vi "Teleop.vi"(10 "Match Info":T1={"Autonomous Elapsed Seconds"=0.0, "TeleOp Elapsed Seconds"=0.0, "Disabled Elapsed Seconds"=0.0, "Visited Autonomous"=FALSE, "Visited TeleOp"=FALSE, "Visited Disabled"=FALSE, "Autonomous Settings"={"Autonomous Style"=enum."Independent", "VI Refnum"=refnum}}, 11 "Call Context":T2) -> ()   [LabVIEW 2016]
doc: "This VI is called for each TeleOp packet received from the DS where the robot is not disabled. It is often used to read from the joysticks and update I/O or to update setpoints for timed control loops. It should complete and return within 20 milliseconds or it may miss DS packets."
uses:
  <vilib>/Rock Robotics/WPI/DriverStation/WPI_DriverStationDerivedRobotMode.ctl
  <vilib>/Rock Robotics/WPI/DriverStation/WPI_DriverStationMatch Info.ctl
  <vilib>/Rock Robotics/WPI/Utilities/WPI_GetSetVariantRefNum.vi
  <vilib>/Rock Robotics/Network Tables/NT Write Boolean Array.vi
  <vilib>/Rock Robotics/Network Tables/NT Write Numeric Array.vi
  <vilib>/Rock Robotics/Network Tables/NT Read Boolean.vi
  <vilib>/Rock Robotics/Network Tables/NT Read Number.vi
  <vilib>/Rock Robotics/Network Tables/NT Write Boolean.vi
  <vilib>/Rock Robotics/Network Tables/NT Write Number.vi
panel:
  out "Difference":dbl(knob) scale=0.0..50.0
  in  "Reset Counters":bool
  out "Right Wheel Sensor Count":dbl
  out "Left Wheel Sensor Count":dbl
  out "Low Switch":bool
  out "High Switch":bool
  out "POT Sensor Meter":dbl(knob) scale=78.0..98.0
  out "POT Sensor Value":dbl
  out "Sample Slider 0":dbl(slide) scale=0.0..5.0
  out "Sample Boolean 1":bool
  out "Sample Boolean 0":bool
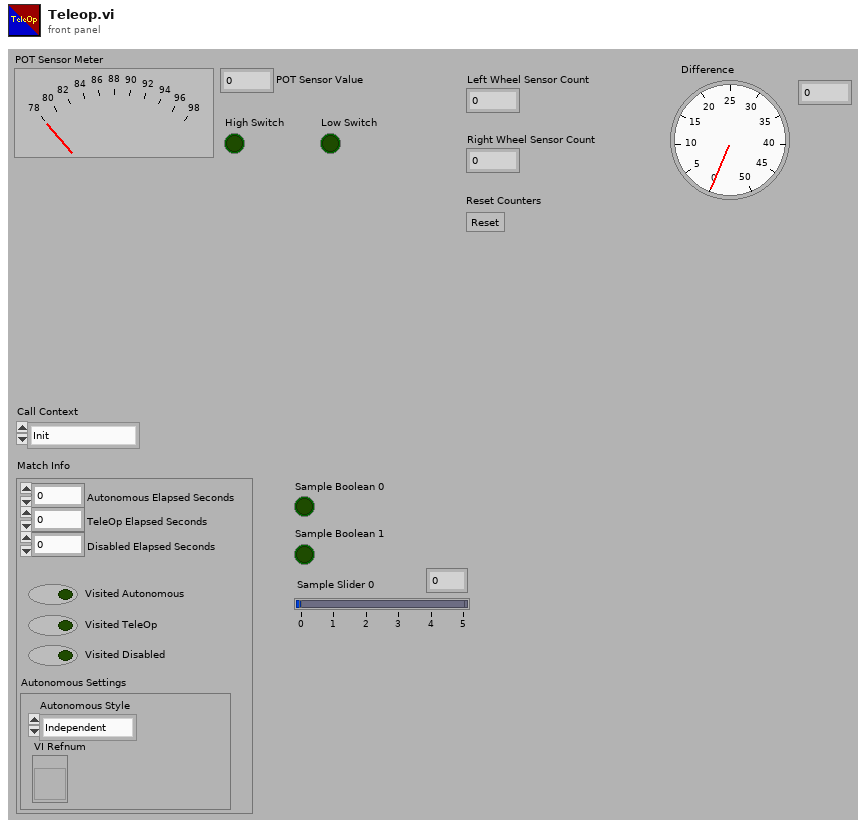
[diagram p1: front panel]
types:
  T1 = typedef "WPI_DriverStationMatch Info.ctl" = cluster{"Autonomous Elapsed Seconds":dbl, "TeleOp Elapsed Seconds":dbl, "Disabled Elapsed Seconds":dbl, "Visited Autonomous":bool, "Visited TeleOp":bool, "Visited Disabled":bool, "Autonomous Settings":cluster{"Autonomous Style":enum16{"Iterative", "Independent"}, "VI Refnum":refnum<vi>}}
  T2 = typedef "WPI_DriverStationDerivedRobotMode.ctl" = enum16{"Init", "Execute", "Stop"}
  T3 = typedef "WPI_JoystickDevRef.ctl" = cluster{"Device":T4}
  T4 = typedef "WPI_JoystickDeviceEnum.ctl" = enum16{"USB 0", "USB 1", "USB 2", "USB 3", "USB 4", "USB 5"}
  T5 = typedef "WPI_SwitchDevRef.ctl" = cluster{"DevStatus":errorcluster, "DIO Channel":T6, "CntIndex":T7, "Normally Closed":bool}
  T6 = typedef "FPGA_DIOChannel.ctl" = enum8{"DIO 0", "DIO 1", "DIO 2", "DIO 3", "DIO 4", "DIO 5", "DIO 6", "DIO 7", "DIO 8", "DIO 9", "DIO MXP 0", "DIO MXP 1", "DIO MXP 2", "DIO MXP 3", "DIO MXP 4", "DIO MXP 5", "DIO MXP 6", "DIO MXP 7", "DIO MXP 8", "DIO MXP 9", "DIO MXP 10", "DIO MXP 11", "DIO MXP 12", "DIO MXP 13", "DIO MXP 14", "DIO MXP 15", "SPI Port CS1", "SPI Port CS2", "SPI Port CS3", "SPI Port MISO", "SPI Port MOSI", "Invalid"}
  T7 = typedef "FPGA_CounterCtrSystemIndex.ctl" = enum8{"Ctr 0", "Ctr 1", "Ctr 2", "Ctr 3", "Ctr 4", "Ctr 5", "Ctr 6", "Ctr 7", "Invalid"}
  T8 = typedef "WPI_PotentiometerDevRef.ctl" = cluster{"DevStatus":errorcluster, "Analog Channel":T9, "Invert Output":bool}
  T9 = typedef "FPGA_AIChannel.ctl" = enum8{"AI 0", "AI 1", "AI 2", "AI 3", "AI MXP 0", "AI MXP 1", "AI MXP 2", "AI MXP 3", "Invalid"}
  T10 = cluster{"Axes[0]":dbl, "Axes[1]":dbl, "Axes[2]":dbl, "Axes[3]":dbl, "Axes[4]":dbl, "Axes[5]":dbl, "Axes[6]":dbl, "Axes[7]":dbl, "Axes[8]":dbl}
  T11 = typedef "WPI_RobotDriveDevRef.ctl" = cluster{"DevStatus":errorcluster, "Motors[]":T12[], "Square Inputs":bool, "Max Output":dbl}
  T12 = typedef "WPI_MotorControlDeviceRef.ctl" = cluster{"DeviceStatus":errorcluster, "Type":T13, "PWM":cluster{"PWM Channel":T14, "DeadBand":T15}, "CAN":cluster{"Device Number":u8, "SetOutput VI Ref":variant, "GetOutput VI Ref":variant, "Enable VI Ref":variant, "Disable VI Ref":variant, "Data":variant}, "Invert":bool}
  T13 = typedef "WPI_MotorControlType.ctl" = enum16{"PWM", "CAN"}
  T14 = typedef "FPGA_DIOPWMChannel.ctl" = enum8{"PWM 0", "PWM 1", "PWM 2", "PWM 3", "PWM 4", "PWM 5", "PWM 6", "PWM 7", "PWM 8", "PWM 9", "PWM MXP 0", "PWM MXP 1", "PWM MXP 2", "PWM MXP 3", "PWM MXP 4", "PWM MXP 5", "PWM MXP 6", "PWM MXP 7", "PWM MXP 8", "PWM MXP 9", "Invalid"}
  T15 = typedef "WPI_PWMDeadband.ctl" = cluster{"Name":string, "maxPositivePwm":i32, "minPositivePwm":i32, "centerPwm":i32, "maxNegativePwm":i32, "minNegativePwm":i32, "angularRange":u16}
  T16 = cluster{"Buttons[0]":bool, "Buttons[1]":bool, "Buttons[2]":bool, "Buttons[3]":bool, "Buttons[4]":bool, "Buttons[5]":bool, "Buttons[6]":bool, "Buttons[7]":bool, "Buttons[8]":bool}
  T17 = typedef "WPI_ServoDeviceRef.ctl" = cluster{"DeviceStatus":errorcluster, "PWM Channel":T14, "DeadBand":T15}
  T18 = typedef "WPI_CounterDevRef.ctl" = cluster{"DevStatus":errorcluster, "CntIndex":T7}
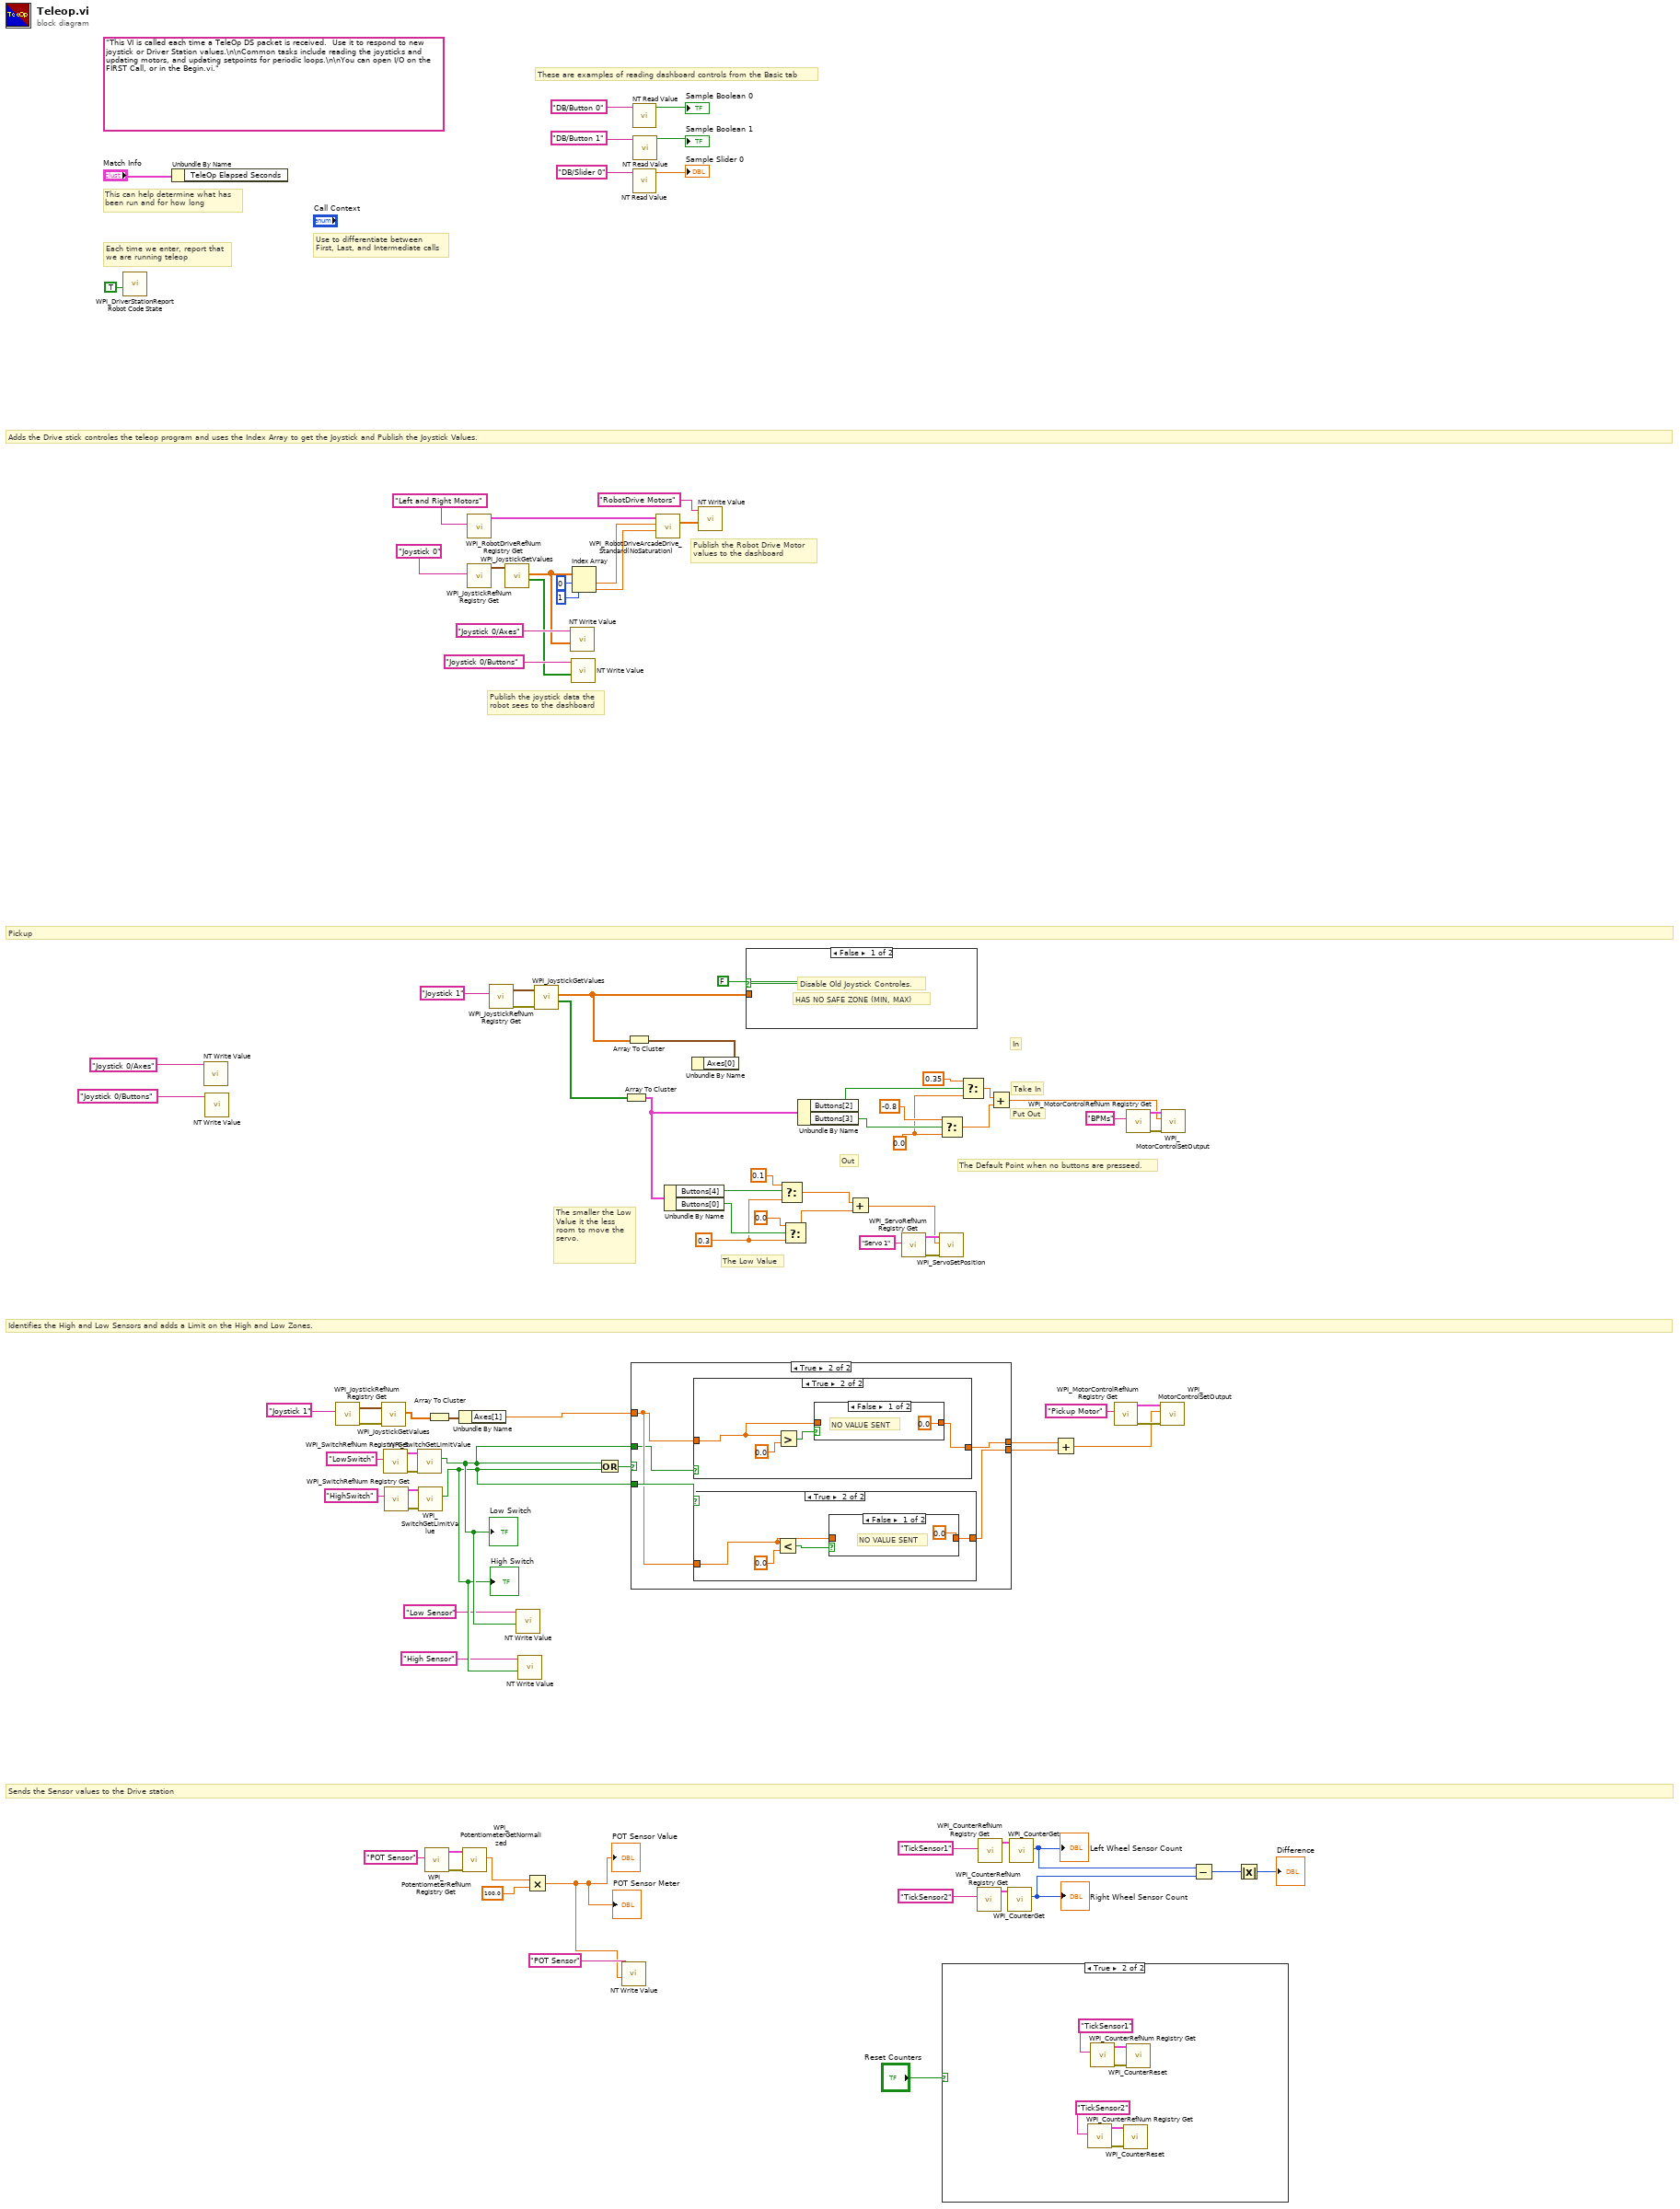
[diagram p0: block diagram]
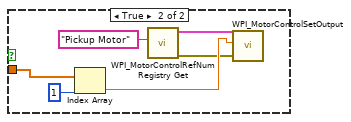
[diagram p3: hidden frame]
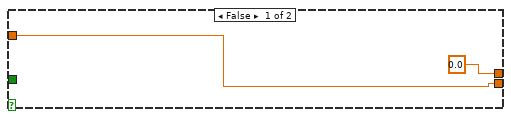
[diagram p4: hidden frame]
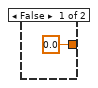
[diagram p5: hidden frame]
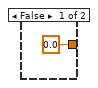
[diagram p7: hidden frame]
diagram:
  w12 = 0.3 ("f")
  w10 = 0.0 ("f")
  (unwired) "This VI is called each time a TeleOp DS packet is received.  Use it to respond to new joystick or Driver Station values.\n\nCommon tasks include reading the joysticks and updating motors, and updating setpoints for periodic loops.\n\nYou can open I/O on the FIRST Call, or in the Begin.vi."
  # "In"
  # "Out"
  # "Adds the Drive stick controles the teleop program and uses the Index Array to get the Joystick and Publish the Joystick Values."
  # "Sends the Sensor values to the Drive station"
  # "Identifies the High and Low Sensors and adds a Limit on the High and Low Zones."
  # "The Default Point when no buttons are presseed."
  # "The smaller the Low Value it the less room to move the servo."
  # "The Low Value"
  # "Put Out"
  # "Take In"
  # "Pickup"
  # "These are examples of reading dashboard controls from the Basic tab"
  # "Publish the Robot Drive Motor\nvalues to the dashboard"
  # "Publish the joystick data the\nrobot sees to the dashboard"
  # "Each time we enter, report that\nwe are running teleop"
  # "Use to differentiate between\nFirst, Last, and Intermediate calls"
  # "This can help determine what has\nbeen run and for how long"
  n1 = call <vilib>:"WPI_DriverStationReport Robot Code State.vi"("TeleOp"=TRUE ("Autonomous")) -> ()  [unwired: 10 in, 1 out]
  n2 = Unbundle By Name("Match Info") -> ()  [unwired: 1 out]
  n3 = call-poly <vilib>:"NT Write Value.vi"("Name"="Joystick 0/Axes") -> ()  [unwired: 10 in, 1 out]
  n4 = call-poly <vilib>:"NT Write Value.vi"("Name"="Joystick 0/Buttons") -> ()  [unwired: 10 in, 1 out]
  n5 = call <vilib>:"WPI_JoystickRefNum Registry Get.vi"("refnum name"="Joystick 1") -> ("error out"=w46:errorcluster, "JoystickDevRef"=w47:T3)  [unwired: 9 in]
  n6 = call <vilib>:"WPI_JoystickGetValues.vi"("error in (no error)"=w46, "JoystickDevRef"=w47) -> ("Axes"=w45:dbl[])  [unwired: 5 in, 4 out]
  n7 = call <vilib>:"WPI_SwitchRefNum Registry Get.vi"("refnum name"="LowSwitch") -> ("error out"=w53:errorcluster, "SwitchDevRef"=w54:T5)  [unwired: 9 in]
  n8 = call <vilib>:"WPI_SwitchRefNum Registry Get.vi"("refnum name"="HighSwitch") -> ("error out"=w50:errorcluster, "SwitchDevRef"=w51:T5)  [unwired: 9 in]
  n9 = call <vilib>:"WPI_SwitchGetLimitValue.vi"("error in (no error)"=w53, "SwitchDevRef"=w54) -> ("Switch Pressed"=w30:bool)  [unwired: 7 in, 2 out]
  "Low Switch" <- w30
  n10 = call <vilib>:"WPI_SwitchGetLimitValue.vi"("error in (no error)"=w50, "SwitchDevRef"=w51) -> ("Switch Pressed"=w29:bool)  [unwired: 7 in, 2 out]
  "High Switch" <- w29
  n11 = call <vilib>:"WPI_PotentiometerRefNum Registry Get.vi"("refnum name"="POT Sensor") -> ("error out"=w34:errorcluster, "PotDevRef"=w33:T8)  [unwired: 9 in]
  n12 = Array To Cluster(array=w45) -> (cluster=w44:T10)
  n13 = Unbundle By Name(w44) -> ("Axes[1]"=w43:dbl)
  n14 = call <vilib>:"WPI_PotentiometerGetNormalized.vi"("error in"=w34, "PotDevRef"=w33) -> ("Normalized Value"=w26:dbl)  [unwired: 7 in, 2 out]
  n15 = call <vilib>:"WPI_RobotDriveRefNum Registry Get.vi"("refnum name"="Left and Right Motors") -> ("RobotDriveDevRef"=w91:T11)  [unwired: 1 in, 9 out]
  n16 = call <vilib>:"WPI_JoystickRefNum Registry Get.vi"("refnum name"="Joystick 0") -> ("JoystickDevRef"=w88:T3)  [unwired: 1 in, 9 out]
  n17 = call <vilib>:"WPI_JoystickRefNum Registry Get.vi"("refnum name"="Joystick 1") -> ("error out"=w70:errorcluster, "JoystickDevRef"=w71:T3)  [unwired: 9 in]
  n18 = call <vilib>:"WPI_JoystickGetValues.vi"("JoystickDevRef"=w88) -> ("Buttons"=w56:bool[], "Axes"=w83:dbl[])  [unwired: 6 in, 3 out]
  n19 = call-poly <vilib>:"NT Write Value.vi"("Boolean"=w30, "Name"="Low Sensor") -> ()  [unwired: 9 in, 1 out]
  n20 = call-poly <vilib>:"NT Write Value.vi"("Boolean"=w29, "Name"="High Sensor") -> ()  [unwired: 9 in, 1 out]
  n21 = Multiply(x=w26, y=100.0) -> (x*y=w24:dbl)
  "POT Sensor Value" <- w24
  "POT Sensor Meter" <- w24
  n22 = call <vilib>:"WPI_JoystickGetValues.vi"("error in (no error)"=w70, "JoystickDevRef"=w71) -> ("Buttons"=w59:bool[], "Axes"=w35:dbl[])  [unwired: 5 in, 3 out]
  n23 = call-poly <vilib>:"NT Write Value.vi"("Numeric Array"=w83, "Name"="Joystick 0/Axes") -> ()  [unwired: 9 in, 1 out]
  n24 = call-poly <vilib>:"NT Write Value.vi"("Boolean Array"=w56, "Name"="Joystick 0/Buttons") -> ()  [unwired: 9 in, 1 out]
  n25 = Index Array(array=w83, index #1=0 ("index"), index #2=1 ("index")) -> (element #1=w90:dbl, element #2=w86:dbl)
  n26 = Or(x=w30, y=w29) -> (x .or. y?=w55:bool)
  n27 = call-poly <vilib>:"NT Write Value.vi"("Numeric"=w24, "Name"="POT Sensor") -> ()  [unwired: 9 in, 1 out]
  n28 = Array To Cluster(array=w59) -> (cluster=w14:T16)
  n29 = Array To Cluster(array=w35) -> (cluster=w58:T10)
  n30 = case shown="True" w55 {
    tunnel: w30 -> [_ w98]
    tunnel: w29 -> [_ w100]
    tunnel: w43 -> [w94 w99]
    tunnel: [0.0 ("Axes[1]") w97] -> w38
    tunnel: [w94 w96] -> w37
    frame False {
    }
    frame True {
      n31 = case shown="True" w98 {
        tunnel: w99 -> [_ w110]
        tunnel: [0.0 ("Axes[1]") w109] -> w97
        frame False {
        }
        frame True {
          n32 = Greater?(x=w110, y=0.0) -> (0:w111:bool)
          n33 = case shown="False" w111 {
            tunnel: [0.0 ("Axes[1]") w114] -> w109
            tunnel: w110 -> [_ w114]
            frame False {
              # "NO VALUE SENT"
            }
            frame True {
            }
          }
        }
      }
      n34 = case shown="True" w100 {
        tunnel: w99 -> [_ w102]
        tunnel: [0.0 ("Axes[1]") w103] -> w96
        frame False {
        }
        frame True {
          n35 = Less?(x=w102, y=0.0) -> (x < y?=w104:bool)
          n36 = case shown="False" w104 {
            tunnel: [0.0 ("Axes[1]") w107] -> w103
            tunnel: w102 -> [_ w107]
            frame False {
              # "NO VALUE SENT"
            }
            frame True {
            }
          }
        }
      }
    }
  }
  n37 = call-poly <vilib>:"NT Read Value.vi"("Name"="DB/Button 0" ("refnum name")) -> ("Boolean"=→"Sample Boolean 0":bool)  [unwired: 9 in, 1 out]
  n38 = call-poly <vilib>:"NT Read Value.vi"("Name"="DB/Slider 0" ("refnum name")) -> ("Numeric"=→"Sample Slider 0":dbl)  [unwired: 9 in, 1 out]
  n39 = call-poly <vilib>:"NT Read Value.vi"("Name"="DB/Button 1" ("refnum name")) -> ("Boolean"=→"Sample Boolean 1":bool)  [unwired: 9 in, 1 out]
  n40 = call <vilib>:"WPI_RobotDriveArcadeDrive_Standard(NoSaturation).vi"("Y axis value"=w86, "X axis value"=w90, "RobotDriveDevRef"=w91) -> ("Motor Values"=w76:dbl[])  [unwired: 1 in, 7 out]
  n41 = Unbundle By Name(w14) -> ("Buttons[4]"=w13:bool, "Buttons[0]"=w18:bool)
  n42 = Unbundle By Name(w58) -> ()  [unwired: 1 out]
  n43 = call-poly <vilib>:"NT Write Value.vi"("Numeric Array"=w76, "Name"="RobotDrive Motors") -> ()  [unwired: 9 in, 1 out]
  n44 = case shown="False" FALSE {
    tunnel: w35 -> [_ w115]
    frame False {
      # "HAS NO SAFE ZONE (MIN, MAX)"
      # "Disable Old Joystick Controles."
    }
    frame True {
      n45 = Index Array(array=w115, index=1) -> (element=w119:dbl)
      n46 = call <vilib>:"WPI_MotorControlRefNum Registry Get.vi"("refnum name"="Pickup Motor") -> ("error out"=w116:errorcluster, "MotorControlDevRef"=w117:T12)  [unwired: 9 in]
      n47 = call <vilib>:"WPI_MotorControlSetOutput.vi"("error in (no error)"=w116, "Output"=w119, "MotorControlDevRef"=w117) -> ()  [unwired: 6 in, 3 out]
    }
  }
  n48 = Select(t=0.1, s=w13, f=w12) -> (s? t:f=w15:dbl)
  n49 = Select(t=0.0, s=w18, f=w12) -> (s? t:f=w17:dbl)
  n50 = Unbundle By Name(w14) -> ("Buttons[2]"=w57:bool, "Buttons[3]"=w11:bool)
  n51 = Add(x=w15, y=w17) -> (x+y=w16:dbl)
  n52 = call <vilib>:"WPI_ServoRefNum Registry Get.vi"("refnum name"="Servo 1") -> ("error out"=w22:errorcluster, "ServoDeviceRef"=w21:T17)  [unwired: 9 in]
  n53 = call <vilib>:"WPI_ServoSetPosition.vi"("error in (no error)"=w22, "Position"=w16, "ServoDeviceRef"=w21) -> ()  [unwired: 7 in, 2 out]
  n54 = Select(t=-0.8, s=w11, f=w10) -> (s? t:f=w63:dbl)
  n55 = case shown="True" "Reset Counters" {
    frame False {
    }
    frame True {
      n56 = call <vilib>:"WPI_CounterRefNum Registry Get.vi"("refnum name"="TickSensor2") -> ("error out"=w125:errorcluster, "CounterDevRef"=w126:T18)  [unwired: 9 in]
      n57 = call <vilib>:"WPI_CounterRefNum Registry Get.vi"("refnum name"="TickSensor1") -> ("error out"=w122:errorcluster, "CounterDevRef"=w123:T18)  [unwired: 9 in]
      n58 = call <vilib>:"WPI_CounterReset.vi"("error in (no error)"=w125, "CounterDevRef in"=w126) -> ()  [unwired: 8 in, 2 out]
      n59 = call <vilib>:"WPI_CounterReset.vi"("error in (no error)"=w122, "CounterDevRef in"=w123) -> ()  [unwired: 8 in, 2 out]
    }
  }
  n60 = Select(t=0.35, s=w57, f=w10) -> (s? t:f=w64:dbl)
  n61 = call <vilib>:"WPI_CounterRefNum Registry Get.vi"("refnum name"="TickSensor2") -> ("CounterDevRef"=w6:T18)  [unwired: 9 in, 1 out]
  n62 = call <vilib>:"WPI_CounterRefNum Registry Get.vi"("refnum name"="TickSensor1") -> ("CounterDevRef"=w8:T18)  [unwired: 9 in, 1 out]
  n63 = Add(x=w64, y=w63) -> (x+y=w62:dbl)
  n64 = call <vilib>:"WPI_CounterGet.vi"("CounterDevRef in"=w6) -> ("Value"=w3:i32)  [unwired: 5 in, 5 out]
  "Right Wheel Sensor Count" <- w3
  n65 = call <vilib>:"WPI_CounterGet.vi"("CounterDevRef in"=w8) -> ("Value"=w4:i32)  [unwired: 5 in, 5 out]
  "Left Wheel Sensor Count" <- w4
  n66 = Add(x=w38, y=w37) -> (x+y=w39:dbl)
  n67 = call <vilib>:"WPI_MotorControlRefNum Registry Get.vi"("refnum name"="Pickup Motor") -> ("error out"=w42:errorcluster, "MotorControlDevRef"=w41:T12)  [unwired: 9 in]
  n68 = call <vilib>:"WPI_MotorControlRefNum Registry Get.vi"("refnum name"="BPMs") -> ("error out"=w68:errorcluster, "MotorControlDevRef"=w69:T12)  [unwired: 9 in]
  n69 = call <vilib>:"WPI_MotorControlSetOutput.vi"("error in (no error)"=w42, "Output"=w39, "MotorControlDevRef"=w41) -> ()  [unwired: 6 in, 3 out]
  n70 = call <vilib>:"WPI_MotorControlSetOutput.vi"("error in (no error)"=w68, "Output"=w62, "MotorControlDevRef"=w69) -> ()  [unwired: 6 in, 3 out]
  n71 = Subtract(x=w4, y=w3) -> (x-y=w2:i32)
  n72 = Absolute Value(x=w2) -> (abs(x)=→"Difference":i32)
